vi "Dashboard Main.vi"() -> ()   [LabVIEW 2013]
uses:
  Target detection/TargetType.ctl
  <vilib>/event_ctls.llb/eventvkey.ctl
  <vilib>/Rock Robotics/WPI/Dashboard/WPI_DashboardLogging Global.vi
  <vilib>/Utility/config.llb/Write Key (String).vi
  <vilib>/Utility/config.llb/Write Key (I32).vi
  <vilib>/Utility/config.llb/NI_LVConfig.lvlib
panel:
  out "Image Message":string="Timeout in Camera Communications"
  in  "Rec Mode":enum32{"Stop", "Record", "Playback"}(radio)
  in  "Dashboard Tab":T1(tab)
  in  "Camera Settings":T2={"Frame Rate"=30, "Compression"=30, "Size"=1} {"Frame Rate" scale=1.0..30.0; "Size" items=["640x480", "320x240", "160x120"]}
  out "MotorSliders R":cluster{"MotorSlide1":dbl, "MotorSlide2":dbl} {"MotorSlide2" scale=-1.0..1.0 scale format="%#_2e"; "MotorSlide1" scale=-1.0..1.0 scale format="%#_2e"}
  out "MotorChart R":cluster{"Numeric":dbl, "Numeric":dbl}(graph)
  out "MotorSliders L":T3 {"MotorSlide4 2" scale=0.0..14.0 scale format="%#_2e"; "MotorSlide2" scale=-1.0..1.0 scale format="%#_2e"; "MotorSlide1" scale=-1.0..1.0 scale format="%#_2e"}
  out "MotorChart L":T4(graph)
  out "JS1 Z":dbl(slide) scale=-1.0..1.0 scale format="%#_2e"
  out "Joystick 1":cluster{"X":dbl, "Y":dbl}[](graph)
  out "JS Buttons 1":T5
  out "JS2 Z":dbl(slide) scale=-1.0..1.0 scale format="%#_2e"
  out "Joystick 2":cluster{"X":dbl, "Y":dbl}[](graph)
  out "JS Buttons 2":T5
  out "Mode":T6(ring)=enum."Auto Disabled"
  out "Camera IP":string
  in  "DB Camera Config":bool
  out "fps":dbl format="%#.1g"
  out "Mbps":dbl format="%#.1g"
  out "Mbps 2":bool
  out "LED 1":bool
  in  "Compressor On":bool
  in  "Slider 1":dbl(slide) scale=0.0..100.0
  out "Mask":T7(plugin-control)
  out "Distances":T9(array[cluster])
  in  "Score Limit":dbl=70.0
  in  "Color Components":T10={"Hue"={110.0, 142.0}, "Sat"={138.0, 255.0}, "Val"={139.0, 198.0}} {"Val" scale=0.0..255.0; "Sat" scale=0.0..255.0; "Hue" scale=0.0..255.0 scale format="%#_3g"}
  in  "Checkbox 2":bool
  in  "Checkbox 1":bool
  in  "Test Slider":dbl(slide) scale=0.0..100.0 scale format="%#_3g"
  in  "On/Off":bool caption="Solenoid"
  in  "Test Name":u16(ring) items=["Select the test to run...", "Example Test", "-------------------------------", "List of tests is built in robot code.", "Replace with your own automated tests."]
  in  "Test Tree":string(tree)
  in  "Motor":cluster{"Value":dbl, "Enable":bool} {"Value" scale=-1.0..1.0 scale format="%#_3g"}
  out "Progress":T11 {"Test Progress" scale=0.0..100.0}
  in  "Rev/Fwd":cluster{"Forward":bool, "Reverse":bool}
  in  "Test Ring":u16(ring) items=["Auto", "Fixed indoor", "Fixed outdoor 1", "Fixed outdoor 2", "Fixed fluorescent 1", "Fixed fluorescent 2", "Hold current"]
  in  "Listbox":i32(listbox)
  out "Tree":string(tree)
  out "Camera Image":T7(plugin-control)
  in  "Enable":bool
  # "Left"
  # "Front"
  # "Right"
  # "Battery"
  # "Customize by placing controls and indicators here and name to\nmatch Dashboard Variables on robot."
  # "This tab is a great place for autonomous settings and validation.\nCustomize by placing controls and indicators here and name to\nmatch Dashboard Variables on robot."
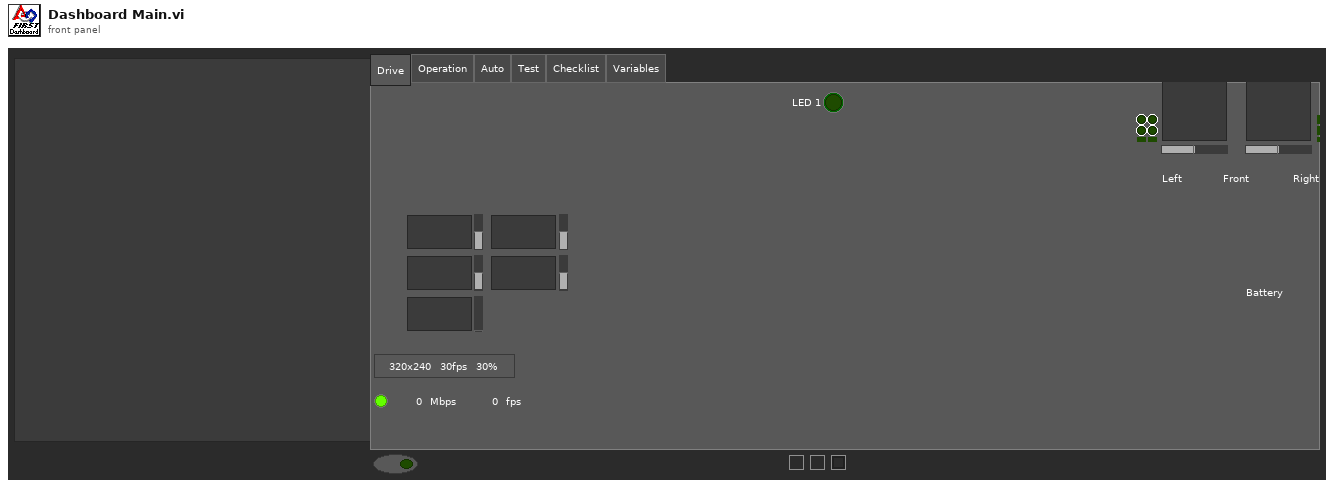
[diagram p1: front panel]
types:
  T1 = enum32{"Drive", "Operation", "Auto", "Test", "Checklist", "Variables"}
  T2 = cluster{"Frame Rate":i32, "Compression":i32, "Size":u16}
  T3 = cluster{"MotorSlide1":dbl, "MotorSlide2":dbl, "MotorSlide4 2":dbl}
  T4 = cluster{"Numeric":dbl, "Numeric":dbl, "Battery":sgl}
  T5 = cluster{bool, bool, bool, bool, bool, bool, bool, bool, bool, bool, bool, bool}
  T6 = enum8{"Tele-Op Disabled", "Tele-Op Enabled", "Auto Disabled", "Auto Enabled", "Test Disabled", "Test Enabled", ""}
  T7 = typedef "IMAQ Image.ctl" = refnum<image>
  T8 = typedef "TargetType.ctl" = enum16{"Not Hot", "Hot"}
  T9 = cluster{"Distance (ft)":dbl, "Target Center (-1 to 1)":cluster{"X":dbl, "Y":dbl}, "Left":bool, "State":T8}[]
  T10 = cluster{"Hue":cluster{dbl, dbl}, "Sat":cluster{dbl, dbl}, "Val":cluster{dbl, dbl}}
  T11 = cluster{"Test Progress":u8, "Test Progress Text":string}
  T12 = typedef "Image Type" = u32
  T13 = cluster{"Horizontal":bool, "Aspect Score":dbl, "Rect Score":dbl, cluster{"Left":dbl, "Top":dbl, "Right":dbl, "Bottom":dbl}, "Equiv H":dbl, "Equiv V":dbl}[]
  T14 = cluster{"Scores":cluster{"Total":dbl, "Left":dbl, "Right":dbl, "Ratio":dbl, "Vertical":dbl, "index":i32, "State":T8}, "Verticals":cluster{"Horizontal?":bool, "Aspect Score":dbl, "Rect Score":dbl, cluster{"Left":dbl, "Top":dbl, "Right":dbl, "Bottom":dbl}, "Equiv H":dbl, "Equiv V":dbl}, "Horizontals":cluster{"Horizontal?":bool, "Aspect Score":dbl, "Rect Score":dbl, cluster{"Left":dbl, "Top":dbl, "Right":dbl, "Bottom":dbl}, "Equiv H":dbl, "Equiv V":dbl}, "Validated":bool}[]
  T15 = cluster{cluster{dbl, dbl}, cluster{dbl, dbl}, cluster{dbl, dbl}}
  T16 = cluster{"Digital Inputs":bool[], "Digital Outputs":bool[]}
  T17 = cluster{"Competition mode":bool, "Robot Link":bool, "Autonomous":bool, "Enabled":bool, "E-Stop":bool, "Simulated":bool, "TestMode":bool, "Docked Window":bool}
  T18 = cluster{"Boolean Array[0]":bool, "Boolean Array[1]":bool, "Boolean Array[2]":bool, "Boolean Array[3]":bool, "Boolean Array[4]":bool, "Boolean Array[5]":bool, "Boolean Array[6]":bool, "Boolean Array[7]":bool, "Boolean Array[8]":bool, "Boolean Array[9]":bool, "Boolean Array[10]":bool, "Boolean Array[11]":bool}
  T19 = typedef "NI_LVConfig.lvlib/Config Data RefNum.ctl" = refnum<k1>
  T20 = typedef "eventvkey.ctl" = enum16{"ASCII", "Enter", "Return", "Shift", "Ctrl", "Alt", "Cmd", "Opt", "Caps", "NumLock", "Clear", "Break", "Up", "Down", "Left", "Right", "Insert", "Delete", "Home", "End", "PageUp", "PageDown", "Escape", "Help", "Pause", "ScrollLock", "F1", "F2", "F3", "F4", "F5", "F6", "F7", "F8", "F9", "F10", "F11", "F12", "F13", "F14", "F15", "F16", "F17", "F18", "F19", "F20", "F21", "F22", "F23", "F24", "Play", "VolumeUp", "VolumeDown", "Mute", "Two Byte Char"}
  T21 = cluster{"Image Size":bool, "Image Type":bool, "Pixel Value":bool, "ROI Information":bool, "Zoom Factor":bool}
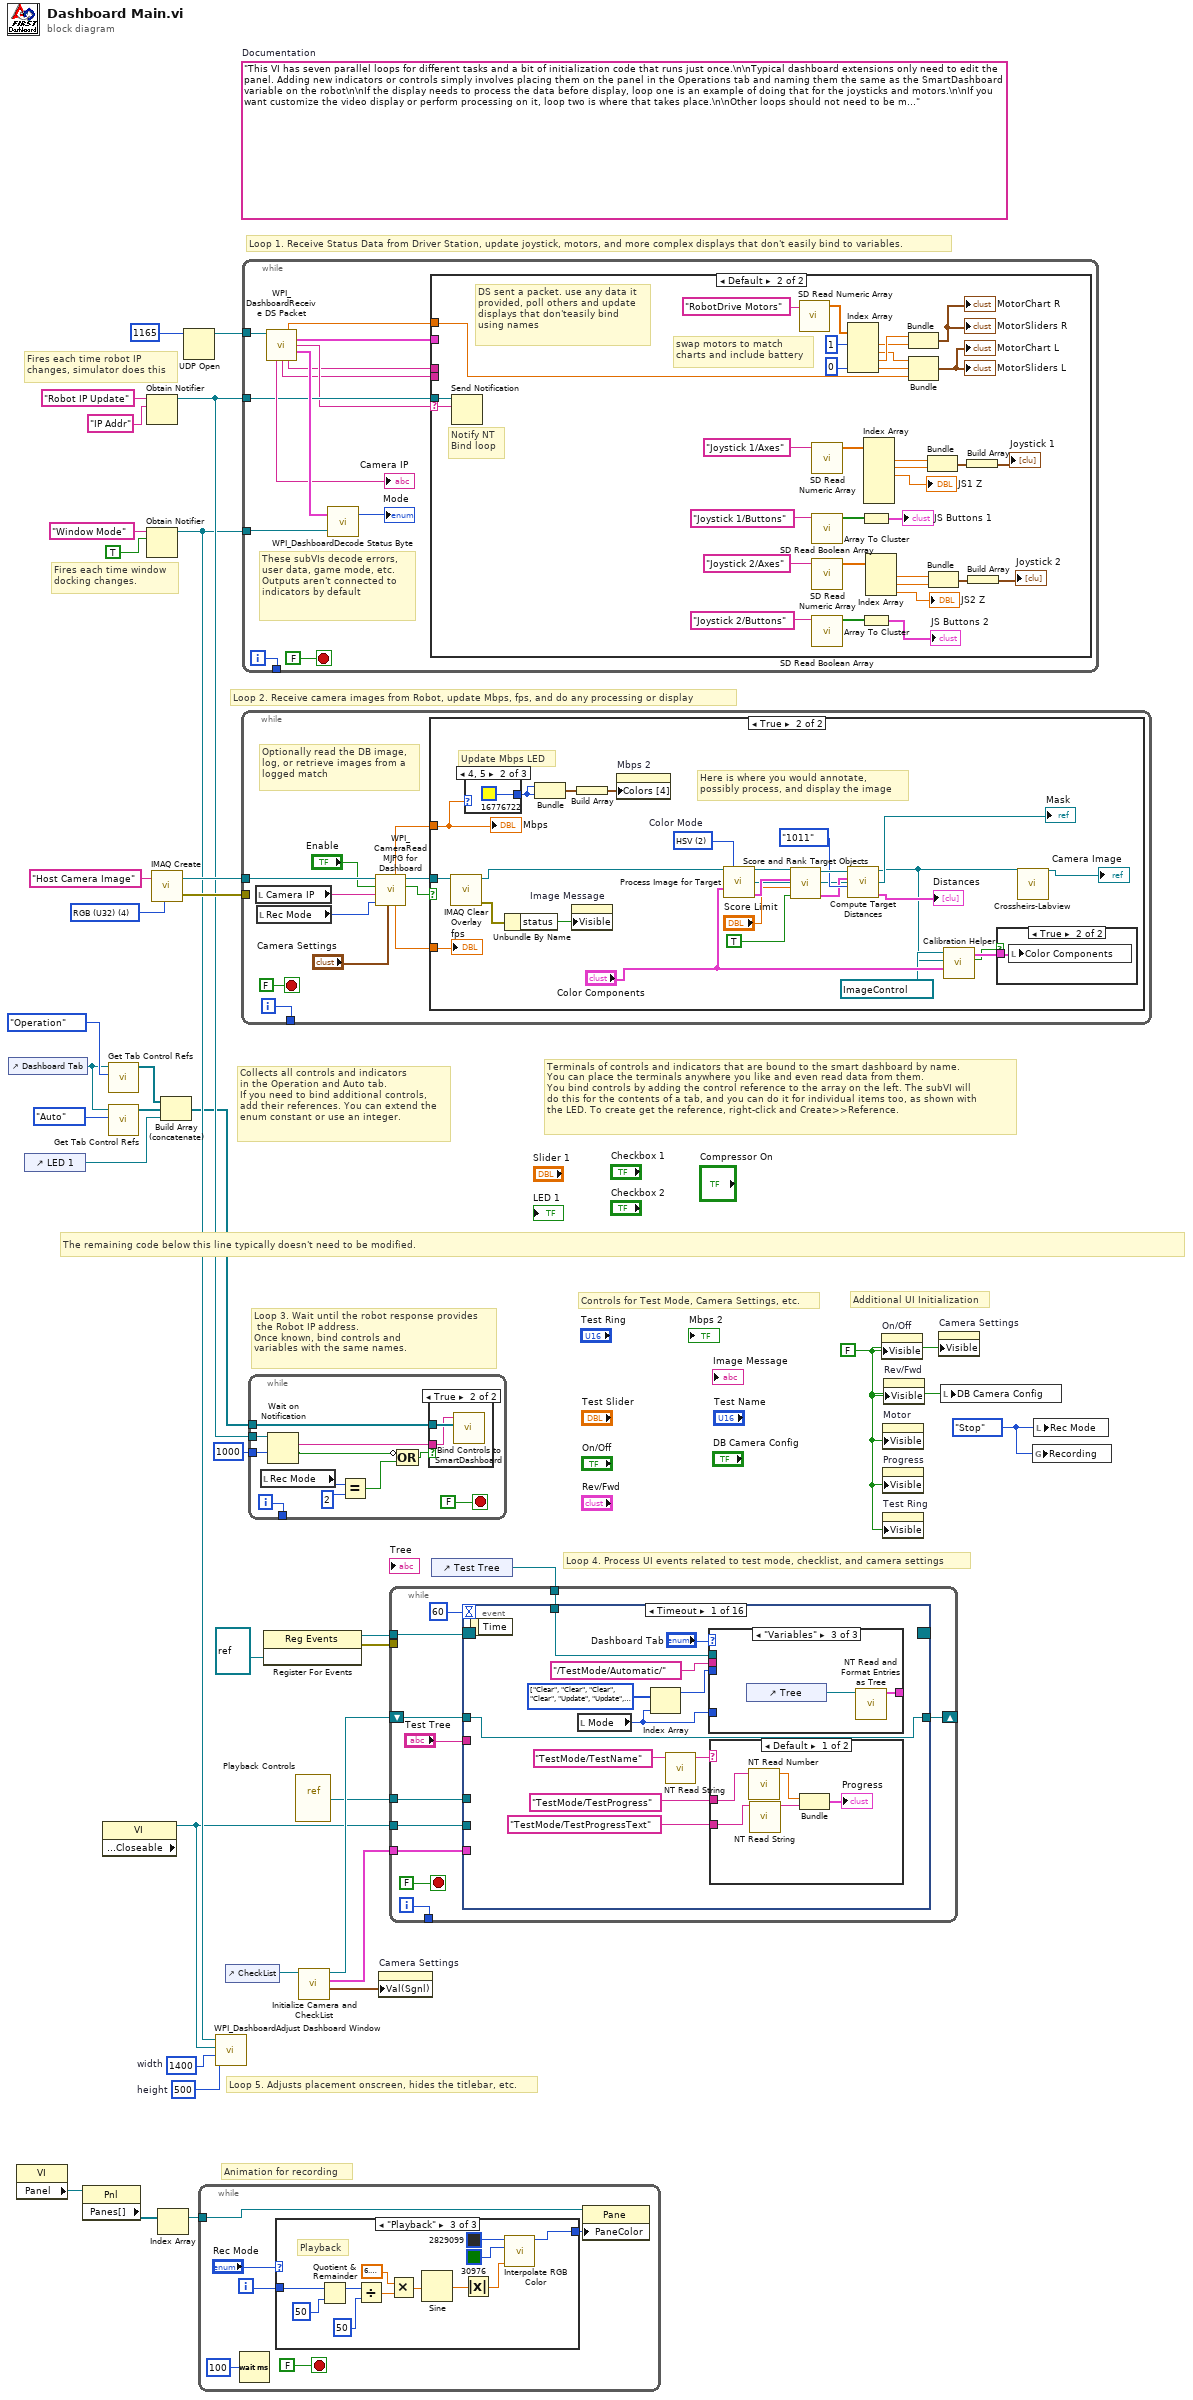
[diagram p0: block diagram]
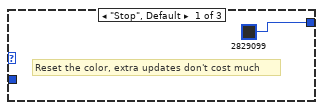
[diagram p2: hidden frame]
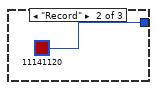
[diagram p3: hidden frame]
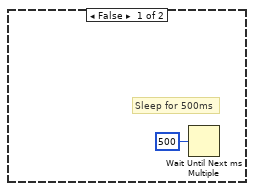
[diagram p5: hidden frame]
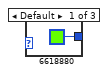
[diagram p7: hidden frame]
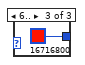
[diagram p8: hidden frame]
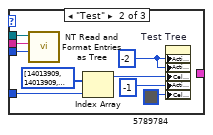
[diagram p10: hidden frame]
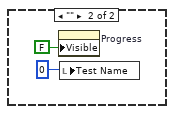
[diagram p11: hidden frame]
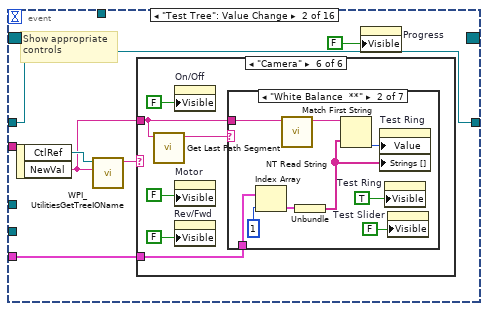
[diagram p12: hidden frame]
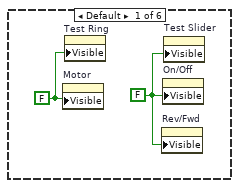
[diagram p13: hidden frame]
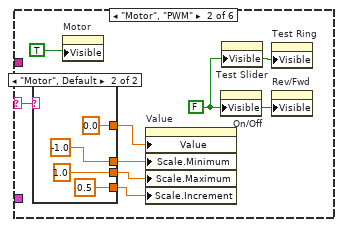
[diagram p14: hidden frame]
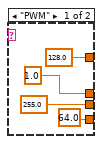
[diagram p15: hidden frame]
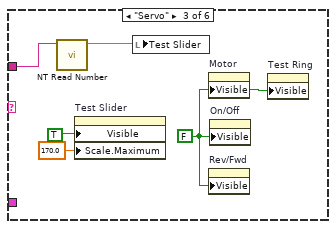
[diagram p16: hidden frame]
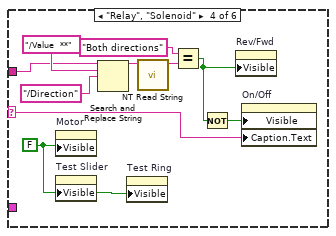
[diagram p17: hidden frame]
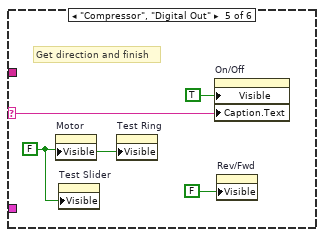
[diagram p18: hidden frame]
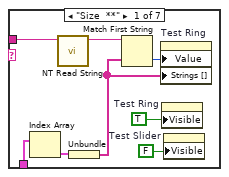
[diagram p19: hidden frame]
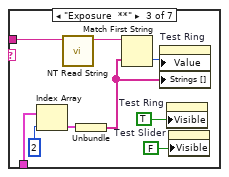
[diagram p20: hidden frame]
diagram:
  w8 = enum32{"Stop", "Record", "Playback"}."Stop" ("Rec Mode")
  w11 = 500  # height
  w12 = 1400  # width
  w25 = FALSE ("Visible")
  (unwired) "This VI has seven parallel loops for different tasks and a bit of initialization code that runs just once.\n\nTypical dashboard extensions only need to edit the panel. Adding new indicators or controls simply involves placing them on the panel in the Operations tab and naming them the same as the SmartDashboard variable on the robot\n\nIf the display needs to process the data before display, loop one is an example of doing that for the joysticks and motors.\n\nIf you want customize the video display or perform processing on it, loop two is where that takes place.\n\nOther loops should not need to be modified. They are pretty standard, and document the task they perform."  # Documentation
  w35 = T12 4 items=["Grayscale (U8)", "Grayscale (I16)", "Grayscale (SGL)", "Complex (CSG)", "RGB (U32)", "HSL (U32)", "RGB (U64)"] ("Image Type")
  # "Controls for Test Mode, Camera Settings, etc."
  # "Additional UI Initialization"
  # "Animation for recording"
  # "Fires each time robot IP\nchanges, simulator does this"
  # "Fires each time window\ndocking changes."
  # "Collects all controls and indicators\nin the Operation and Auto tab.\nIf you need to bind additional controls,\nadd their references. You can extend the\nenum constant or use an integer."
  # "The remaining code below this line typically doesn't need to be modified."
  # "Loop 4. Process UI events related to test mode, checklist, and camera settings"
  # "Terminals of controls and indicators that are bound to the smart dashboard by name.\nYou can place the terminals anywhere you like and even read data from them.\nYou bind controls by adding the control reference to the array on the left. The subVI will\ndo this for the contents of a tab, and you can do it for individual items too, as shown with\nthe LED. To create get the reference, right-click and Create>>Reference."
  # "Loop 3. Wait until the robot response provides\n the Robot IP address.\nOnce known, bind controls and\nvariables with the same names."
  # "Loop 5. Adjusts placement onscreen, hides the titlebar, etc."
  # "Loop 1. Receive Status Data from Driver Station, update joystick, motors, and more complex displays that don't easily bind to variables."
  # "Loop 2. Receive camera images from Robot, update Mbps, fps, and do any processing or display"
  n1 = control-ref of="Dashboard Tab"() -> (w6:refnum<vi>)
  n2 = property class="VI"() -> ("Panel"=w19:refnum<vi>)  [unwired: 2 in, 2 out]
  n3 = control-ref of="LED 1"() -> (w1:refnum<vi>)
  n4 = property class="Pnl"(reference=w19) -> ("Panes[]"=w20:refnum<vi>[])  [unwired: 1 in, 2 out]
  n5 = property class="VI" props=["Front Panel.Closeable"]() -> (reference out=w7:refnum<vi>)  [unwired: 2 in, 2 out]
  n6 = call <vilib>:"Get Tab Control Refs.vi"("Page Index"=T1."Operation" ("Dashboard Tab"), "TabControl in"=w6) -> ("ControlsOnPage"=w4:refnum<vi>[])  [unwired: 9 in]
  n7 = call <vilib>:"Get Tab Control Refs.vi"("Page Index"=T1."Auto" ("Dashboard Tab"), "TabControl in"=w6) -> ("ControlsOnPage"=w5:refnum<vi>[])  [unwired: 9 in]
  n8 = Obtain Notifier(name (unnamed)="Robot IP Update", notification data type="IP Addr" ("name (unnamed)")) -> (notifier out=w29:refnum<notifier>)  [unwired: 2 in, 2 out]
  n9 = Obtain Notifier(name (unnamed)="Window Mode", notification data type=TRUE) -> (notifier out=w10:refnum<notifier>)  [unwired: 2 in, 2 out]
  n10 = call "IMAQ Create"("Image Name"="Host Camera Image", "Image Type"=w35) -> ("New Image"=w33:T7, "error out"=w32:errorcluster)  [unwired: 2 in, 1 out]
  n11 = Index Array(array=w20) -> (element=w18:refnum<vi>)  [unwired: 1 in]
  n12 = Build Array (concatenate)(w4, w5, w1) -> (w3:refnum<vi>[])
  n13 = UDP Open(11:u16 1165 ("port")) -> (port=w36:refnum<k16>)  [unwired: 2 in, 4 out]
  n14 = while {
    tunnel: w18 -> [w39]
    i -> [w42]
    stop <- FALSE stop-if-true
    n15 = Wait (ms)(milliseconds to wait=u32 100) -> ()  [unwired: 1 out]
    n16 = case shown="\"Playback\"" "Rec Mode" {
      tunnel: w42 -> [_ _ w57]
      tunnel: [u32 2829099 ("Base Color") u32 11141120 ("Target Color") w46] -> w38
      frame "Stop", Default {
        # "Reset the color, extra updates don't cost much"
      }
      frame "Record" {
      }
      frame "Playback" {
        # "Playback"
        n17 = Quotient & Remainder(x=w57, y=u32 50 ("milliseconds to wait")) -> (x-y*floor(x/y)=w53:u32)  [unwired: 1 out]
        n18 = Divide(x=w53, y=u32 50 ("milliseconds to wait")) -> (x/y=w50:dbl)
        n19 = Multiply(x=6.283185307179586, y=w50) -> (x*y=w55:dbl)
        n20 = Sine(x=w55) -> (sin(x)=w54:dbl)
        n21 = Absolute Value(x=w54) -> (abs(x)=w47:dbl)
        n22 = call "Interpolate RGB Color.vi"("Proportion"=w47, "Target Color"=u32 30976, "Base Color"=u32 2829099) -> ("Result Color"=w46:u32)  [unwired: 8 in]
      }
    }
    n23 = property class="Pane"(reference=w39, "PaneColor"=w38) -> ()  [unwired: 1 in, 2 out]
  }
  n24 = call <vilib>:"WPI_DashboardAdjust Dashboard Window.vi"("height"=w11, "width"=w12, "reference in"=w7, "Notifier in"=w10) -> ()  [unwired: 8 in]
  n25 = control-ref of="CheckList"() -> (w9:refnum<vi>)
  n26 = while {
    tunnel: w33 -> [w66]
    tunnel: w32 -> [_]
    tunnel: [w67] -> _
    i -> [w67]
    stop <- FALSE stop-if-true
    # "Optionally read the DB image,\nlog, or retrieve images from a\nlogged match"
    n27 = local read "Camera IP"() -> (w59:string)
    n28 = local read "Rec Mode"() -> (w58:enum32{"Stop", "Record", "Playback"})
    n29 = call <vilib>:"WPI_CameraRead MJPG for Dashboard.vi"("Camera Settings"="Camera Settings", "Rec Mode"=w58, "Camera IP"=w59, "Enable"="Enable", "Refnum in"=w66) -> ("Active"=w63:bool, "Refnum out"=w65:T7, "FPS"=w62:dbl, "Bandwidth (Mbps)"=w61:dbl)  [unwired: 3 in]
    n30 = case shown="True" w63 {
      tunnel: w65 -> [_ w89]
      tunnel: w61 -> [_ w88]
      tunnel: w62 -> [_ w87]
      frame False {
        # "Sleep for 500ms"
        n31 = Wait Until Next ms Multiple(millisecond multiple=u32 500) -> ()  [unwired: 1 out]
      }
      frame True {
        w72 = u16 2 items=["RGB", "HSL", "HSV", "HSI"]  # Color Mode
        # "Here is where you would annotate,\npossibly process, and display the image"
        # "Update Mbps LED"
        n32 = call "IMAQ Clear Overlay"("Image"=w89) -> ("error out"=w93:errorcluster, "Image Out"=w86:T7)  [unwired: 2 in, 7 out]
        n33 = case shown="4, 5" w88 {
          tunnel: [u32 6618880 ("Color Box") u32 16776722 ("Color Box") u32 16716800 ("Color Box")] -> w90
          frame Default {
          }
          frame 4, 5 {
          }
          frame 6.. {
          }
        }
        n34 = Unbundle By Name(w93) -> ("status"=w94:bool)
        n35 = Bundle("Color Box"=w90, "Color Box"=w90) -> (w92:cluster{"Color Box":u32, "Color Box":u32})  [unwired: 1 out]
        n36 = property on="Image Message" class="Str"("Visible"=w94) -> ()  [unwired: 2 in, 2 out]
        n37 = Build Array(w92) -> (w91:cluster{"Color Box":u32, "Color Box":u32}[])
        n38 = property on="Mbps 2" class="Bool (strict)"("Colors [4]"=w91) -> ()  [unwired: 2 in, 2 out]
        n39 = call "Process Image for Target.vi"("Src Image"=w86, "Color Mode"=w72, "Color Components"="Color Components") -> ("Src Image Out"=w85:T7, "Threshold"=→"Mask":T7, "Particles"=w81:T13)  [unwired: 10 in]
        n40 = call "Score and Rank Target Objects.vi"("Annotate"=TRUE, "Score Limit"="Score Limit", "Particles"=w81, "Image in"=w85) -> ("Target Info"=w76:T14, "Annotated Image"=w84:T7)  [unwired: 6 in]
        n41 = call "Compute Target Distances.vi"("Camera Type"=enum16{"206", "1011", "1013"}."1011", "Target Info"=w76, "Image in"=w84) -> ("Distances"=→"Distances":T9, "Image out"=w71:T7)  [unwired: 6 in, 1 out]
        n42 = call "Calibration Helper.vi"("Color Components"="Color Components", "Image"=w71, "Image Ctl Refnum"=refnum<vi> refnum) -> ("Changed"=w74:bool, "output color"=w82:T15)  [unwired: 7 in]
        n43 = case shown="True" w74 {
          tunnel: w82 -> [_ w95]
          frame False {
          }
          frame True {
            n44 = local write "Color Components"(w95) -> ()
          }
        }
        n45 = call "Crossheirs-Labview.vi"("Image In"=w71) -> ("Image Out"=→"Camera Image":T7)  [unwired: 25 in, 1 out]
        "Mbps" <- w88
        "fps" <- w87
      }
    }
  }
  n46 = while {
    tunnel: w36 -> [w109]
    tunnel: w29 -> [w104]
    tunnel: w10 -> [w108]
    tunnel: [w105] -> _
    i -> [w105]
    stop <- FALSE stop-if-true
    # "These subVIs decode errors, user data, game mode, etc.\nOutputs aren't connected to indicators by default"
    n47 = call <vilib>:"WPI_DashboardReceive DS Packet.vi"("Recv Socket"=w109) -> ("Battery"=w99:sgl, "Driver Station"=w100:T16, "Robot IP Address"=w103:string, "Status"=w110:T17, "Camera IP Address"=→"Camera IP":string, "Low Priority User Data"=w102:string, "High Priority User Data"=w101:string)  [unwired: 1 in, 7 out]
    n48 = call <vilib>:"WPI_DashboardDecode Status Byte.vi"("Window Mode Notifier"=w108, "Status"=w110) -> ("Mode"=→"Mode":T6)  [unwired: 1 out]
    n49 = case shown="Default" w103 {
      selector: w103 -> [_ w122]
      tunnel: w104 -> [_ w123]
      tunnel: w102 -> [_ _]
      tunnel: w101 -> [_ _]
      tunnel: w100 -> [_ _]
      tunnel: w99 -> [_ w121]
      frame "0.0.0.0" {
        # "DS not sending packets, or no robot exists yet.\nDon't poll the variables"
      }
      frame Default {
        # "Notify NT\nBind loop"
        # "DS sent a packet. use any data it\nprovided, poll others and update\ndisplays that don'teasily bind\nusing names"
        # "swap motors to match\ncharts and include battery"
        n50 = Send Notification(notification=w122, notifier=w123) -> ()  [unwired: 1 in, 2 out]
        n51 = call <vilib>:"SD Read Numeric Array.vi"("Name"="RobotDrive Motors") -> ("Numeric Array"=w120:dbl[])  [unwired: 8 in, 2 out]
        n52 = call <vilib>:"SD Read Numeric Array.vi"("Name"="Joystick 1/Axes") -> ("Numeric Array"=w139:dbl[])  [unwired: 8 in, 2 out]
        n53 = call <vilib>:"SD Read Boolean Array.vi"("Name"="Joystick 1/Buttons") -> ("Boolean Array"=w141:bool[])  [unwired: 8 in, 2 out]
        n54 = call <vilib>:"SD Read Numeric Array.vi"("Name"="Joystick 2/Axes") -> ("Numeric Array"=w133:dbl[])  [unwired: 8 in, 2 out]
        n55 = call <vilib>:"SD Read Boolean Array.vi"("Name"="Joystick 2/Buttons") -> ("Boolean Array"=w132:bool[])  [unwired: 8 in, 2 out]
        n56 = Index Array(array=w120, index #1=1, index #4=0) -> (element #1=w116:dbl, element #2=w115:dbl, element #3=w117:dbl, element #4=w112:dbl)  [unwired: 2 in]
        n57 = Array To Cluster(array=w141) -> (cluster=→"JS Buttons 1":T18)
        n58 = Array To Cluster(array=w132) -> (cluster=→"JS Buttons 2":T18)
        n59 = Index Array(array=w139) -> (element #1=w136:dbl, element #2=w137:dbl, element #3=→"JS1 Z":dbl)  [unwired: 6 in, 3 out]
        n60 = Index Array(array=w133) -> (element #1=w128:dbl, element #2=w127:dbl, element #3=→"JS2 Z":dbl)  [unwired: 3 in]
        n61 = Bundle("Numeric"=w117, "Numeric"=w116) -> (→"MotorChart R" →"MotorSliders R":cluster{"Numeric":dbl, "Numeric":dbl})  [unwired: 1 in]
        n62 = Bundle("Numeric"=w115, "Numeric"=w112, "Battery"=w121) -> (→"MotorChart L" →"MotorSliders L":T4)  [unwired: 1 in]
        n63 = Bundle("Numeric"=w136, "Numeric"=w137) -> (w135:cluster{"Numeric":dbl, "Numeric":dbl})  [unwired: 1 in]
        n64 = Bundle("Numeric"=w128, "Numeric"=w127) -> (w129:cluster{"Numeric":dbl, "Numeric":dbl})  [unwired: 1 in]
        n65 = Build Array(w135) -> (→"Joystick 1":cluster{"Numeric":dbl, "Numeric":dbl}[])
        n66 = Build Array(w129) -> (→"Joystick 2":cluster{"Numeric":dbl, "Numeric":dbl}[])
      }
    }
  }
  n67 = while {
    tunnel: w3 -> [w155]
    tunnel: w29 -> [w153]
    tunnel: [w151] -> _
    tunnel: u32 1000 ("milliseconds to wait") -> [w150]
    i -> [w151]
    stop <- FALSE stop-if-true
    n68 = local read "Rec Mode"() -> (w146:enum32{"Stop", "Record", "Playback"})
    n69 = Wait on Notification(notifier=w153, timeout in ms (-1)=w150) -> (notification=w152:string, timed out?=w148:bool)  [unwired: 2 in, 2 out]
    n70 = Equal?(x=w146, y=u16 2 ("Rec Mode")) -> (x = y?=w147:bool)
    n71 = Compound Arithmetic op=OR(invert w148, w147) -> (w149:bool)
    n72 = case shown="True" w149 {
      tunnel: w155 -> [_ w157]
      tunnel: w152 -> [_ w156]
      frame False {
      }
      frame True {
        n73 = call <vilib>:"Bind Controls to SmartDashboard.vi"("Bound Control Refs"=w157, "Server IP Address"=w156) -> ()  [unwired: 10 in]
      }
    }
  }
  n74 = register-events(refnum<vi> refnum) -> (reference out=w16:refnum<event-registration>, error out=w15:errorcluster)  [unwired: 2 in]
  n75 = vi-ref "Playback Controls.vi"() -> (w17:refnum<vi>)
  n76 = call "Initialize Camera and CheckList.vi"("ListBox in"=w9) -> ("Cluster"=w23:cluster{"value":i32, "value":i32, "index":i32}, "Array"=w24:cluster{string[]}[], "File Refnum"=w22:T19)  [unwired: 8 in]
  n77 = property on="Camera Settings" class="Clust (strict)"("Val(Sgnl)"=w23) -> ()  [unwired: 2 in, 2 out]
  n78 = control-ref of="Test Tree"() -> (w21:refnum<vi>)
  n79 = while {
    tunnel: w24 -> [w165]
    shift-right: [w164] -> _
    shift-left: w22 -> [w163]
    tunnel: [w162] -> _
    tunnel: w21 -> [w161]
    tunnel: w17 -> [w160]
    tunnel: w16 -> [w159]
    tunnel: w15 -> [_]
    tunnel: w7 -> [w158]
    i -> [w162]
    stop <- FALSE stop-if-true
    n80 = event shown="[0] Timeout" {
      selector: w159 -> [_ _ _ _ _ _ _ _ _ _ _ _ _ _ _ _]
      dyn-events: [_ _ _ _ _ _ _ _ _ _ _ _ _ w403 _ _] -> _
      timeout: u32 60 ("milliseconds to wait") -> [_ _ _ _ _ _ _ _ _ _ _ _ _ _ _ _]
      tunnel: w161 -> [w175 _ _ _ _ _ _ _ _ _ _ _ _ _ _ _]
      tunnel: "Test Tree" -> [_ _ _ _ _ _ _ _ w372 w380 w382 w386 w394 _ _ _]
      tunnel: w165 -> [_ w199 _ _ _ _ w336 w366 _ _ _ _ _ _ _ _]
      tunnel: [w169 w198 w297 w302 w310 w322 w335 w359 w371 w378 w381 w385 w393 w405 w419 w420] -> w164
      tunnel: w163 -> [w169 w198 w297 w302 w310 w322 w334 w359 w371 w378 w381 w385 w393 w405 w419 w420]
      tunnel: w160 -> [_ _ _ _ _ _ _ _ _ _ _ _ _ w406 _ w423]
      tunnel: w158 -> [_ _ _ _ _ _ _ _ _ _ _ _ _ w401 _ _]
      event Timeout {
        w174 = enum16{"Update", "Clear"}[] [enum."Clear", enum."Clear", enum."Clear", enum."Clear", enum."Update", enum."Update", enum."Clear"] items=["Update", "Clear"]
        n81 = event-data() -> ()  [unwired: 1 in, 1 out]
        n82 = local read "Mode"() -> (w172:T6)
        n83 = Index Array(array=w174, index=w172) -> (element=w173:enum16{"Update", "Clear"})
        n84 = call <vilib>:"NT Read String.vi"("Name"="TestMode/TestName") -> ("String"=w178:string)  [unwired: 9 in, 1 out]
        n85 = case shown="\"Variables\"" "Dashboard Tab" {
          tunnel: w175 -> [_ w188 _]
          tunnel: "/TestMode/Automatic/" ("Name Pattern") -> [_ w187 _]
          tunnel: w173 -> [_ w186 _]
          tunnel: w172 -> [_ w184 _]
          tunnel: [_ _ w190] -> _
          frame "Operation", Default {
          }
          frame "Test" {
            w183 = -2 ("Active Item:Row Number")
            n86 = call <vilib>:"NT Read and Format Entries as Tree.vi"("Operation"=w186, "Name Pattern"=w187, "Tree Refnum"=w188) -> ()  [unwired: 7 in, 2 out]
            n87 = Index Array(array=u32[] [14013909, 14013909, 14013909, 14013909, 14013909, 16777215, 14013909], index=w184) -> (element=w182:u32)
            n88 = property on="Test Tree" class="Tree (strict)"("Active Item Row Number"=w183, "ActiveColNum"=w183, "CellBG"=w182, "Active Item Row Number"=-1 ("Active Item:Row Number"), "CellBG"=u32 5789784 ("Color Box")) -> ()  [unwired: 2 in, 2 out]
          }
          frame "Variables" {
            n89 = control-ref of="Tree"() -> (w189:refnum<vi>)
            n90 = call <vilib>:"NT Read and Format Entries as Tree.vi"("Tree Refnum"=w189) -> ("Formatted Strings"=w190:cluster{"Name":string, "Value":string}[])  [unwired: 9 in, 1 out]
          }
        }
        n91 = case shown="Default" w178 {
          tunnel: "TestMode/TestProgress" ("Name") -> [w192 _]
          tunnel: "TestMode/TestProgressText" ("Name") -> [w191 _]
          frame Default {
            n92 = call <vilib>:"NT Read Number.vi"("Name"=w192) -> ("Numeric"=w193:dbl)  [unwired: 9 in, 1 out]
            n93 = call <vilib>:"NT Read String.vi"("Name"=w191) -> ("String"=w194:string)  [unwired: 9 in, 1 out]
            n94 = Bundle("Numeric"=w193, "String"=w194) -> (→"Progress":cluster{"Numeric":dbl, "String":string})  [unwired: 1 in]
          }
          frame "" {
            n95 = property on="Progress" class="Clust (strict)"("Visible"=FALSE) -> ()  [unwired: 2 in, 2 out]
            n96 = local write "Test Name"(u16 0) -> ()
          }
        }
      }
      event "Test Tree": Value Change {
        # "Show appropriate\ncontrols"
        n97 = event-data() -> ("CtlRef"=w202:refnum<vi>, "NewVal"=w200:string)  [unwired: 1 in]
        n98 = call <vilib>:"WPI_UtilitiesGetTreeIOName.vi"("NewVal"=w200, "TreeControl in"=w202) -> ("I/O Name"=w203:string)  [unwired: 9 in]
        n99 = case shown="\"Camera\"" w203 {
          selector: w203 -> [_ w210 _ w228 w237 _]
          tunnel: w200 -> [_ _ w225 w227 _ w244]
          tunnel: w199 -> [_ _ _ _ _ w243]
          frame Default {
            w205 = FALSE ("Visible")
            w204 = FALSE ("Visible")
            n100 = property on="Motor" class="Clust (strict)"("Visible"=w204) -> ()  [unwired: 2 in, 2 out]
            n101 = property on="Test Ring" class="Ring (strict)"("Visible"=w204) -> ()  [unwired: 2 in, 2 out]
            n102 = property on="Rev/Fwd" class="Clust (strict)"("Visible"=w205) -> ()  [unwired: 2 in, 2 out]
            n103 = property on="On/Off" class="Bool (strict)"("Visible"=w205) -> ()  [unwired: 2 in, 2 out]
            n104 = property on="Test Slider" class="Slide (strict)"("Visible"=w205) -> ()  [unwired: 2 in, 2 out]
          }
          frame "Motor", "PWM" {
            w211 = FALSE ("Visible")
            n105 = case shown="\"Motor\", Default" w210 {
              tunnel: [1.0 ("Value") -1.0 ("Value")] -> w209
              tunnel: [255.0 ("Value") 1.0 ("Value")] -> w208
              tunnel: [128.0 ("Value") 0.0 ("Value")] -> w207
              tunnel: [64.0 ("Value") 0.5 ("Value")] -> w206
              frame "PWM" {
              }
              frame "Motor", Default {
              }
            }
            n106 = property on="Motor" class="Clust (strict)"("Visible"=TRUE) -> ()  [unwired: 2 in, 2 out]
            n107 = property on="Value" class="Slide (strict)"("Value"=w207, "Scale.Minimum"=w209, "Scale.Maximum"=w208, "Scale.Increment"=w206) -> ()  [unwired: 2 in, 2 out]
            n108 = property on="On/Off" class="Bool (strict)"("Visible"=w211) -> ()  [unwired: 2 in, 2 out]
            n109 = property on="Test Slider" class="Slide (strict)"("Visible"=w211) -> ()  [unwired: 2 in, 2 out]
            n110 = property on="Test Ring" class="Ring (strict)"("Visible"=w211) -> ()  [unwired: 2 in, 2 out]
            n111 = property on="Rev/Fwd" class="Clust (strict)"("Visible"=w211) -> ()  [unwired: 2 in, 2 out]
          }
          frame "Servo" {
            w223 = FALSE ("Visible")
            n112 = call <vilib>:"NT Read Number.vi"("Name"=w225) -> ("Numeric"=w224:dbl)  [unwired: 9 in, 1 out]
            n113 = property on="Test Slider" class="Slide (strict)"("Visible"=TRUE, "Scale.Maximum"=170.0 ("Scale.Range:Maximum")) -> ()  [unwired: 2 in, 2 out]
            n114 = local write "Test Slider"(w224) -> ()
            n115 = property on="Motor" class="Clust (strict)"("Visible"=w223) -> ()  [unwired: 2 in, 2 out]
            n116 = property on="Rev/Fwd" class="Clust (strict)"("Visible"=w223) -> ()  [unwired: 2 in, 2 out]
            n117 = property on="On/Off" class="Bool (strict)"("Visible"=w223) -> ()  [unwired: 2 in, 2 out]
            n118 = property on="Test Ring" class="Ring (strict)"("Visible"=w223) -> ()  [unwired: 2 in, 2 out]
          }
          frame "Relay", "Solenoid" {
            w226 = FALSE ("Visible")
            n119 = property on="Motor" class="Clust (strict)"("Visible"=w226) -> ()  [unwired: 2 in, 2 out]
            n120 = property on="Test Slider" class="Slide (strict)"("Visible"=w226) -> ()  [unwired: 2 in, 2 out]
            n121 = Search and Replace String(input string=w227, search string="/Value  **", replace string="/Direction") -> (result string=w233:string)  [unwired: 5 in, 3 out]
            n122 = property on="Test Ring" class="Ring (strict)"("Visible"=w226) -> ()  [unwired: 2 in, 2 out]
            n123 = call <vilib>:"NT Read String.vi"("Name"=w233) -> ("String"=w231:string)  [unwired: 9 in, 1 out]
            n124 = Equal?(x="Both directions", y=w231) -> (x = y?=w229:bool)
            n125 = Not(x=w229) -> (.not. x?=w230:bool)
            n126 = property on="Rev/Fwd" class="Clust (strict)"("Visible"=w229) -> ()  [unwired: 2 in, 2 out]
            n127 = property on="On/Off" class="Bool (strict)"("Visible"=w230, "Caption.Text"=w228) -> ()  [unwired: 2 in, 2 out]
          }
          frame "Compressor", "Digital Out" {
            w236 = FALSE ("Visible")
            # "Get direction and finish"
            n128 = property on="Motor" class="Clust (strict)"("Visible"=w236) -> ()  [unwired: 2 in, 2 out]
            n129 = property on="Test Slider" class="Slide (strict)"("Visible"=w236) -> ()  [unwired: 2 in, 2 out]
            n130 = property on="Test Ring" class="Ring (strict)"("Visible"=w236) -> ()  [unwired: 2 in, 2 out]
            n131 = property on="On/Off" class="Bool (strict)"("Visible"=TRUE, "Caption.Text"=w237) -> ()  [unwired: 2 in, 2 out]
            n132 = property on="Rev/Fwd" class="Clust (strict)"("Visible"=FALSE) -> ()  [unwired: 2 in, 2 out]
          }
          frame "Camera" {
            n133 = call <vilib>:"Get Last Path Segment.vi"("String in"=w244) -> ("String out"=w245:string)  [unwired: 10 in]
            n134 = property on="On/Off" class="Bool (strict)"("Visible"=FALSE) -> ()  [unwired: 2 in, 2 out]
            n135 = property on="Motor" class="Clust (strict)"("Visible"=FALSE) -> ()  [unwired: 2 in, 2 out]
            n136 = property on="Rev/Fwd" class="Clust (strict)"("Visible"=FALSE) -> ()  [unwired: 2 in, 2 out]
            n137 = case shown="\"White Balance  **\"" w245 {
              tunnel: w244 -> [w251 w260 w269 w278 w287 _ w293]
              tunnel: w243 -> [w249 w257 w266 w275 w284 _ _]
              frame "Size  **" {
                n138 = Index Array(array=w249) -> (element=w248:cluster{string[]})  [unwired: 1 in]
                n139 = call <vilib>:"NT Read String.vi"("Name"=w251) -> ("String"=w250:string)  [unwired: 9 in, 1 out]
                n140 = Unbundle(w248) -> (w246:string[])
                n141 = Match First String(2:w246, 3:w250) -> (0:w247:i32)  [unwired: 1 out]
                n142 = property on="Test Ring" class="Ring (strict)"("Value"=w247, "Strings []"=w246) -> ()  [unwired: 2 in, 2 out]
                n143 = property on="Test Ring" class="Ring (strict)"("Visible"=TRUE) -> ()  [unwired: 2 in, 2 out]
                n144 = property on="Test Slider" class="Slide (strict)"("Visible"=FALSE) -> ()  [unwired: 2 in, 2 out]
              }
              frame "White Balance  **" {
                n145 = Index Array(array=w257, index=1) -> (element=w258:cluster{string[]})
                n146 = call <vilib>:"NT Read String.vi"("Name"=w260) -> ("String"=w259:string)  [unwired: 9 in, 1 out]
                n147 = Unbundle(w258) -> (w255:string[])
                n148 = Match First String(2:w255, 3:w259) -> (0:w254:i32)  [unwired: 1 out]
                n149 = property on="Test Ring" class="Ring (strict)"("Value"=w254, "Strings []"=w255) -> ()  [unwired: 2 in, 2 out]
                n150 = property on="Test Ring" class="Ring (strict)"("Visible"=TRUE) -> ()  [unwired: 2 in, 2 out]
                n151 = property on="Test Slider" class="Slide (strict)"("Visible"=FALSE) -> ()  [unwired: 2 in, 2 out]
              }
              frame "Exposure  **" {
                n152 = Index Array(array=w266, index=2) -> (element=w267:cluster{string[]})
                n153 = call <vilib>:"NT Read String.vi"("Name"=w269) -> ("String"=w268:string)  [unwired: 9 in, 1 out]
                n154 = Unbundle(w267) -> (w263:string[])
                n155 = Match First String(2:w263, 3:w268) -> (0:w264:i32)  [unwired: 1 out]
                n156 = property on="Test Ring" class="Ring (strict)"("Value"=w264, "Strings []"=w263) -> ()  [unwired: 2 in, 2 out]
                n157 = property on="Test Ring" class="Ring (strict)"("Visible"=TRUE) -> ()  [unwired: 2 in, 2 out]
                n158 = property on="Test Slider" class="Slide (strict)"("Visible"=FALSE) -> ()  [unwired: 2 in, 2 out]
              }
              frame "Exposure Priority  **" {
                n159 = Index Array(array=w275, index=3) -> (element=w276:cluster{string[]})
                n160 = call <vilib>:"NT Read String.vi"("Name"=w278) -> ("String"=w277:string)  [unwired: 9 in, 1 out]
                n161 = Unbundle(w276) -> (w272:string[])
                n162 = Match First String(2:w272, 3:w277) -> (0:w273:i32)  [unwired: 1 out]
                n163 = property on="Test Ring" class="Ring (strict)"("Value"=w273, "Strings []"=w272) -> ()  [unwired: 2 in, 2 out]
                n164 = property on="Test Ring" class="Ring (strict)"("Visible"=TRUE) -> ()  [unwired: 2 in, 2 out]
                n165 = property on="Test Slider" class="Slide (strict)"("Visible"=FALSE) -> ()  [unwired: 2 in, 2 out]
              }
              frame "Color Enable  **" {
                n166 = Index Array(array=w284, index=4) -> (element=w285:cluster{string[]})
                n167 = call <vilib>:"NT Read String.vi"("Name"=w287) -> ("String"=w286:string)  [unwired: 9 in, 1 out]
                n168 = Unbundle(w285) -> (w281:string[])
                n169 = Match First String(2:w281, 3:w286) -> (0:w282:i32)  [unwired: 1 out]
                n170 = property on="Test Ring" class="Ring (strict)"("Value"=w282, "Strings []"=w281) -> ()  [unwired: 2 in, 2 out]
                n171 = property on="Test Ring" class="Ring (strict)"("Visible"=TRUE) -> ()  [unwired: 2 in, 2 out]
                n172 = property on="Test Slider" class="Slide (strict)"("Visible"=FALSE) -> ()  [unwired: 2 in, 2 out]
              }
              frame Default {
                n173 = property on="Test Ring" class="Ring (strict)"("Visible"=FALSE) -> ()  [unwired: 2 in, 2 out]
                n174 = property on="Test Slider" class="Slide (strict)"("Visible"=FALSE) -> ()  [unwired: 2 in, 2 out]
              }
              frame "Brightness  **", "Color Level  **", "Compression  **", "FPS  **", "Sharpness  **" {
                n175 = call <vilib>:"NT Read Number.vi"("Name"=w293) -> ("Numeric"=w292:dbl)  [unwired: 9 in, 1 out]
                n176 = local write "Test Slider"(w292) -> ()
                n177 = property on="Test Slider" class="Slide (strict)"("Visible"=TRUE, "Scale.Maximum"=100.0 ("Scale.Range:Maximum")) -> ()  [unwired: 2 in, 2 out]
                n178 = property on="Test Ring" class="Ring (strict)"("Visible"=FALSE) -> ()  [unwired: 2 in, 2 out]
              }
            }
          }
        }
        n179 = property on="Progress" class="Clust (strict)"("Visible"=FALSE) -> ()  [unwired: 2 in, 2 out]
      }
      event "Test Name": Mouse Enter {
        # "Populate the ring with the list of tests"
        n180 = event-data() -> ()  [unwired: 1 in, 1 out]
        n181 = call <vilib>:"NT Read String Array.vi"("Name"="TestMode/TestList") -> ("String Array"=w301:string[])  [unwired: 9 in, 1 out]
        n182 = Build Array (concatenate)("Select the test to run...", w301) -> (w300:string[])
        n183 = property on="Test Name" class="Ring (strict)"("Strings []"=w300) -> ()  [unwired: 2 in, 2 out]
      }
      event "Test Name": Value Change {
        w303 = FALSE ("Visible")
        # "Tell the robot the test name to run"
        n184 = event-data() -> ("NewVal"=w307:u16)  [unwired: 1 in]
        n185 = property on="Test Name" class="Ring (strict)"() -> ("Strings []"=w308:string[])  [unwired: 2 in, 2 out]
        n186 = local write "Progress"(T11 {"Test Progress"=0, "Test Progress Text"=""} ("Progress")) -> ()
        n187 = Index Array(array=w308, index=w307) -> (element=w306:string)
        n188 = call <vilib>:"NT Write String.vi"("String"=w306, "Name"="TestMode/TestName") -> ()  [unwired: 9 in, 1 out]
        n189 = property on="Progress" class="Clust (strict)"("Visible"=TRUE) -> ()  [unwired: 2 in, 2 out]
        n190 = property on="Motor" class="Clust (strict)"("Visible"=w303) -> ()  [unwired: 2 in, 2 out]
        n191 = property on="Test Slider" class="Slide (strict)"("Visible"=w303) -> ()  [unwired: 2 in, 2 out]
        n192 = property on="On/Off" class="Bool (strict)"("Visible"=w303) -> ()  [unwired: 2 in, 2 out]
        n193 = property on="Rev/Fwd" class="Clust (strict)"("Visible"=w303) -> ()  [unwired: 2 in, 2 out]
        n194 = property on="Test Ring" class="Ring (strict)"("Visible"=w303) -> ()  [unwired: 2 in, 2 out]
      }
      event "Listbox": Double Click {
        n195 = event-data() -> ("PlatMods.Shift"=w311:bool, "Row"=w313:i32)  [unwired: 1 in]
        n196 = case shown="True" w311 {
          tunnel: w313 -> [w317 _]
          tunnel: 1 -> [w316 _]
          frame False {
            n197 = property on="Listbox" class="LstBox (strict)"() -> ("Item Symbols"=w315:i32[])  [unwired: 2 in, 2 out]
            n198 = Replace Array Subset(array=w315, new element=w316, index=w317) -> (w314:i32[])
            n199 = property on="Listbox" class="LstBox (strict)"("Item Symbols"=w314) -> ()  [unwired: 2 in, 2 out]
          }
          frame True {
            w318 = 0 ("Top Row")
            n200 = property on="Listbox" class="LstBox (strict)"() -> ("Number of Rows"=w320:u32)  [unwired: 2 in, 2 out]
            n201 = Initialize Array(0, w320) -> (w319:i32[])
            n202 = property on="Listbox" class="LstBox (strict)"("Top Row"=w318, "Value"=w318, "Item Symbols"=w319) -> ()  [unwired: 2 in, 2 out]
          }
        }
      }
      event "Listbox": Key Down {
        n203 = event-data() -> ("VKey"=w324:T20)  [unwired: 1 in]
        n204 = case shown="\"Left\", \"Right\"" w324 {
          selector: w324 -> [w329 _]
          tunnel: eventvkey."Left" ("VKey") -> [w327 _]
          frame "Left", "Right" {
            n205 = Equal?(x=w327, y=w329) -> (x = y?=w328:bool)
            n206 = Select(t=0, s=w328, f=1) -> (s? t:f=w330:i32)
            n207 = property on="Listbox" class="LstBox (strict)"() -> ("Item Symbols"=w333:i32[])  [unwired: 2 in, 2 out]
            n208 = Replace Array Subset(array=w333, new element=w330, index="Listbox") -> (w332:i32[])
            n209 = property on="Listbox" class="LstBox (strict)"("Item Symbols"=w332) -> ()  [unwired: 2 in, 2 out]
          }
          frame Default {
          }
        }
      }
      event "DB Camera Config": Value Change {
        n210 = event-data() -> ("NewVal"=w337:bool)  [unwired: 1 in]
        n211 = case shown="False" w337 {
          tunnel: w336 -> [w346 _]
          tunnel: [w339 w357] -> w335
          tunnel: w334 -> [w338 w357]
          frame False {
            w353 = "Camera"
            w356 = FALSE ("Visible")
            n212 = local read "Camera Settings"() -> (w345:T2)
            n213 = Index Array(array=w346) -> (element=w349:cluster{string[]})  [unwired: 1 in]
            n214 = Unbundle(w345) -> ("Frame Rate"=w344:i32, "Compression"=w343:i32, "Size"=w347:u16)
            n215 = Unbundle(w349) -> (w348:string[])
            n216 = Index Array(array=w348, index=w347) -> (element=w342:string)
            n217 = call-poly <vilib>:"Write Key.vi"("section"=w353, "value"=w342, "key"="Size", "refnum"=w338) -> ("refnum out"=w355:T19)  [unwired: 2 in, 5 out]
            n218 = call-poly <vilib>:"Write Key.vi"("section"=w353, "value"=w344, "key"="FrameRate", "refnum"=w355) -> ("refnum out"=w354:T19)  [unwired: 1 in, 6 out]
            n219 = property on="Camera Settings" class="Clust (strict)"("Visible"=w356) -> ()  [unwired: 2 in, 2 out]
            n220 = local write "DB Camera Config"(w356) -> ()
            n221 = call-poly <vilib>:"Write Key.vi"("section"=w353, "value"=w343, "key"="Compression", "refnum"=w354) -> ("refnum out"=w340:T19)  [unwired: 1 in, 6 out]
            n222 = call <vilib>:"Close Config Data.vi"("refnum"=w340) -> ("file path"=w341:path)  [unwired: 2 in, 8 out]
            n223 = call <vilib>:"Open Config Data.vi"("configuration file path"=w341) -> ("refnum"=w339:T19)  [unwired: 8 in, 2 out]
          }
          frame True {
            n224 = property on="Camera Settings" class="Clust (strict)"("Visible"=TRUE) -> ()  [unwired: 2 in, 2 out]
          }
        }
      }
      event "Camera Settings": Value Change {
        n225 = event-data() -> ("NewVal"=w370:T2)  [unwired: 1 in]
        n226 = Index Array(array=w366) -> (element=w365:cluster{string[]})  [unwired: 1 in]
        n227 = Unbundle(w370) -> ("Frame Rate"=w361:i32, "Compression"=w360:i32, "Size"=w363:u16)
        n228 = Unbundle(w365) -> (w364:string[])
        n229 = Index Array(array=w364, index=w363) -> (element=w362:string)
        n230 = Format Into String(format string="%s   %dfps   %d%%", w362, w361, w360) -> (resulting string=w367:string)  [unwired: 2 in, 1 out]
        n231 = Build Array(w367) -> (w368:string[])
        n232 = property on="DB Camera Config" class="Bool (strict)"("Strings [4]"=w368) -> ()  [unwired: 2 in, 2 out]
      }
      event "Motor.Enable": Value Change {
        n233 = event-data() -> ("NewVal"=w376:bool)  [unwired: 1 in]
        n234 = Unbundle("Motor") -> ("Value"=w375:dbl)  [unwired: 1 out]
        n235 = Select(t=w375, s=w376, f=0.0) -> (s? t:f=w373:dbl)
        n236 = call <vilib>:"NT Write Number.vi"("Numeric"=w373, "Name"=w372) -> ()  [unwired: 9 in, 1 out]
      }
      event "Test Slider": Value Change {
        n237 = event-data() -> ("NewVal"=w379:dbl)  [unwired: 1 in]
        n238 = call <vilib>:"NT Write Number.vi"("Numeric"=w379, "Name"=w380) -> ()  [unwired: 9 in, 1 out]
      }
      event "On/Off": Value Change {
        n239 = event-data() -> ("NewVal"=w384:bool)  [unwired: 1 in]
        n240 = Boolean To (0,1)(Boolean=w384) -> (0, 1=w383:i16)
        n241 = call <vilib>:"NT Write Number.vi"("Numeric"=w383, "Name"=w382) -> ()  [unwired: 9 in, 1 out]
      }
      event "Rev/Fwd": Value Change {
        n242 = event-data() -> ("NewVal.Forward"=w392:bool, "NewVal.Reverse"=w391:bool)  [unwired: 1 in]
        n243 = Boolean To (0,1)(Boolean=w392) -> (0, 1=w388:i16)
        n244 = Boolean To (0,1)(Boolean=w391) -> (0, 1=w390:i16)
        n245 = Negate(x=w390) -> (-x=w389:i16)
        n246 = Add(x=w388, y=w389) -> (x+y=w387:i16)
        n247 = call <vilib>:"NT Write Number.vi"("Numeric"=w387, "Name"=w386) -> ()  [unwired: 9 in, 1 out]
      }
      event "Test Ring": Value Change {
        n248 = event-data() -> ("NewVal"=w396:u16)  [unwired: 1 in]
        n249 = property on="Test Ring" class="Ring (strict)"() -> ("Strings []"=w397:string[])  [unwired: 2 in, 2 out]
        n250 = Index Array(array=w397, index=w396) -> (element=w395:string)
        n251 = call <vilib>:"NT Write String.vi"("String"=w395, "Name"=w394) -> ()  [unwired: 9 in, 1 out]
      }
      event "Rec Mode": Value Change {
        # "Update globals for recording mode and path to read log from.\nClear when logging and let NetworkTables set path for vision to\nuse."
        n252 = event-data() -> ("NewVal"=w407:enum32{"Stop", "Record", "Playback"})  [unwired: 1 in]
        n253 = global write "WPI_DashboardLogging Global.vi" "Logging Filename"(path "") -> ()
        n254 = case shown="\"Stop\", \"Record\"" w407 {
          tunnel: w406 -> [_ w409 w417]
          tunnel: [_ _ w416] -> w403
          tunnel: [_ _ w415] -> _
          tunnel: w401 -> [_ _ w413]
          tunnel: cluster{i32, i32} {-250, 170} -> [_ _ w412]
          tunnel: [_ _ T21 {"Image Size"=TRUE, "Image Type"=TRUE, "Pixel Value"=TRUE, "ROI Information"=TRUE, "Zoom Factor"=FALSE} ("Image Information Shown:All Elements")] -> w399
          tunnel: [_ _ TRUE ("Zoom Factor")] -> w398
          frame Default {
          }
          frame "Stop", "Record" {
            # "Place Window too"
            n255 = invoke class="VI" method="FP.Close"(reference=w409) -> (reference out=w408:refnum<vi>)  [unwired: 2 in, 2 out]
            n256 = invoke class="VI" method="Abort VI"(reference=w408) -> ()  [unwired: 2 in, 3 out]
          }
          frame "Playback" {
            n257 = call "Open Playback Panel.vi"("Offset"=w412, "DB VI Ref"=w413, "Playback in"=w417) -> ("Playback out"=w414:refnum<vi>)  [unwired: 8 in]
            n258 = register-events(w414) -> (reference out=w416:refnum<event-registration>, error out=w415:errorcluster)  [unwired: 2 in]
          }
        }
        n259 = global write "WPI_DashboardLogging Global.vi" "Recording"(w407) -> ()
        n260 = property on="Camera Image" class="ImageControl"("Image Information Shown"=w399, "Image Information Visible"=w398) -> ()  [unwired: 2 in, 2 out]
        n261 = call <vilib>:"WPI_DashboardNT Log FieldName Cache.vi"("Operation"=enum16{"Lookup/Add", "Index", "Clear"}."Clear") -> ()  [unwired: 8 in, 3 out]
      }
      event Panel Close {
        w418 = enum32{"Stop", "Record", "Playback"}."Stop" ("Rec Mode")
        n262 = event-data() -> ()  [unwired: 1 in, 4 out]
        n263 = local write "Rec Mode"(w418) -> ()
        n264 = global write "WPI_DashboardLogging Global.vi" "Recording"(w418) -> ()
      }
      event Panel Close {
        # "Abort playback window and ourself"
        n265 = event-data() -> ()  [unwired: 1 in, 4 out]
        n266 = invoke class="VI" method="FP.Close"(reference=w423) -> (reference out=w422:refnum<vi>)  [unwired: 2 in, 2 out]
        n267 = invoke class="VI" method="Abort VI"(reference=w422) -> (error out=w421:errorcluster)  [unwired: 2 in, 2 out]
        n268 = invoke class="VI" method="Abort VI"(error in=w421) -> ()  [unwired: 2 in, 3 out]
      }
    }
  }
  n269 = property on="On/Off" class="Bool (strict)"("Visible"=w25) -> ()  [unwired: 2 in, 2 out]
  n270 = property on="Motor" class="Clust (strict)"("Visible"=w25) -> ()  [unwired: 2 in, 2 out]
  n271 = property on="Progress" class="Clust (strict)"("Visible"=w25) -> ()  [unwired: 2 in, 2 out]
  n272 = property on="Test Ring" class="Ring (strict)"("Visible"=w25) -> ()  [unwired: 2 in, 2 out]
  n273 = property on="Rev/Fwd" class="Clust (strict)"("Visible"=w25) -> ()  [unwired: 2 in, 2 out]
  n274 = property on="Camera Settings" class="Clust (strict)"("Visible"=w25) -> ()  [unwired: 2 in, 2 out]
  n275 = local write "DB Camera Config"(w25) -> ()
  n276 = global write "WPI_DashboardLogging Global.vi" "Recording"(w8) -> ()
  n277 = local write "Rec Mode"(w8) -> ()
